vi "Edgertronic-Commands_buttons.vi"(3 "error in":errorcluster, 4 "Controls":T1, 5 "URL":string="192.168.1.101") -> (0 "error out":errorcluster, 2 "data out":string="HTTP/1.0 200 OK\r\nContent-Type: text/html; charset=utf-8\r\nContent-Length: 313\r\nConnection: close\r\nDate: Tue, 16 Jun 2015 13:54:12 GMT\r\nServer: lighttpd/1.4.11 (edgertonic slow motion camera)\r\n\r\n{\"build_date\": \"20150112\", \"sw_build_date\": \"20140911165611\", \"fpga_initialized\": 1, \"hardware_revision\": 6, \"model_number\": 1, \"home_dir\": \"/home/root/ss-web\", \"ir_filter\": 1, \"mac_addr\": \"00:1B:C5:09:61:4D\", \"serial_console_enabled\": false, \"serial_number\": 333, \"fpga_version\": 70, \"hardware_configuration\": 1}")   [LabVIEW 2015]
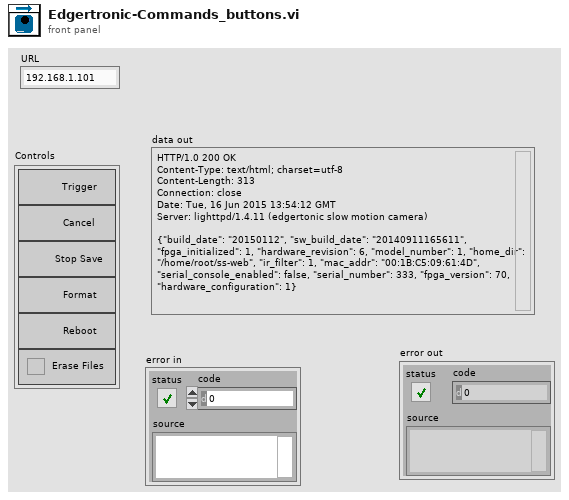
[diagram p1: front panel]
types:
  T1 = cluster{"Trigger":bool, "Cancel":bool, "Stop Save":bool, "Format":bool, "Reboot":bool, "Trash":bool}
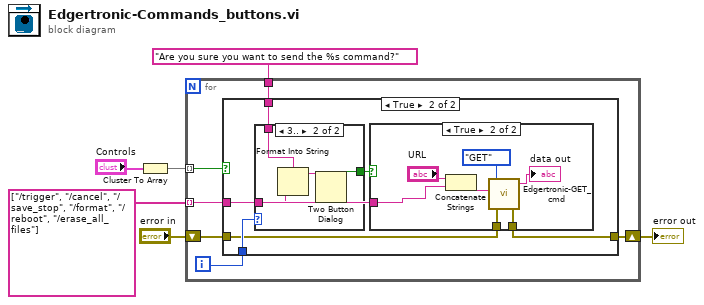
[diagram p0: block diagram]
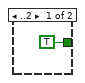
[diagram p4: hidden frame]
diagram:
  n1 = Cluster To Array(cluster="Controls") -> (array=w5:bool[])
  n2 = for {
    tunnel: w5 -> [w12] mode=indexing
    tunnel: string[] ["/trigger", "/cancel", "/save_stop", "/format", "/reboot", "/erase_all_files"] -> [w11] mode=indexing
    tunnel: "Are you sure you want to send the %s command?" ("GET Cmd") -> [w9]
    shift-right: [w7] -> w2
    shift-left: "error in" -> [w8]
    i -> [w10]
    n3 = case shown="True" w12 {
      tunnel: w11 -> [_ w17]
      tunnel: w10 -> [_ w19]
      tunnel: w9 -> [_ w18]
      tunnel: w8 -> [w13 w15]
      tunnel: [w13 w14] -> w7
      frame False {
      }
      frame True {
        n4 = case shown="3.." w19 {
          tunnel: w18 -> [_ w32]
          tunnel: w17 -> [_ w31]
          tunnel: [TRUE ("T button?") w29] -> w16
          frame ..2 {
          }
          frame 3.. {
            n5 = Format Into String(format string=w32, w31) -> (resulting string=w30:string)  [unwired: 2 in, 1 out]
            n6 = Two Button Dialog(message=w30) -> (T button?=w29:bool)  [unwired: 2 in]
          }
        }
        n7 = case shown="True" w16 {
          tunnel: w17 -> [_ w23]
          tunnel: w15 -> [w20 w26]
          tunnel: [w20 w25] -> w14
          frame False {
          }
          frame True {
            n8 = Concatenate Strings("URL", w23) -> (w22:string)
            n9 = call "Edgertronic-GET_cmd.vi"("error in (no error)"=w26, "URL"=w22, "Type"=enum16{"GET", "POST"}."GET") -> ("error out"=w25:errorcluster, "Connection Info"=→"data out":string)  [unwired: 1 in, 1 out]
          }
        }
      }
    }
  }
  "error out" <- w2
